vi "Initialize Control.vi"(8 "error in (no error)":errorcluster, 11 "ScrollZoomGraphChart in":refnum<class "ScrollZoomGraphChart.lvclass">=refnum) -> (0 "error out":errorcluster, 3 "ScrollZoomGraphChart out":refnum<class "ScrollZoomGraphChart.lvclass">)   [LabVIEW 2023, in "ScrollZoomGraphChart.lvclass"]
doc: "The <b>Initialize VI</b> is a dynamic dispatch VI that must be overwritten in every QControl Class. It must <b>Call Parent Method</b> so that it recursively calls the initialize routine all of the way up the inheritance hierarchy. \n\nThe top most call is to the <b>Initialize Control VI</b> in Control.lvclass. This is the VI that starts the <b>Event Handler VI</b> if there was one overwritten in the QControl.\n<b> </b> <b> </b>\n©2016 Q Software Innovations, LLC (QSI)\nwritten by Quentin Alldredge\nproduced in LabVIEW 2015\n\nsupport@qsoftwareinnovations.com\nwww.qsoftwareinnovations.com\n\nAll rights reserved.\n\nRedistribution and use in source and binary forms, with or without modification, are permitted provided that the following conditions are met:\n\n * Redistributions of source code must retain the above copyright notice, this list of conditions and the following disclaimer.\n * Redistributions in binary form must reproduce the above copyright notice, this list of conditions and the following disclaimer in the documentation and/or other materials provided with the distribution.\n * Neither the name of Q Software Innovations, LLC. nor the names of its contributors may be used to endorse or promote products derived from this software without specific prior written permission.\n\nTHIS SOFTWARE IS PROVIDED BY THE COPYRIGHT HOLDERS AND CONTRIBUTORS \"AS IS\" AND ANY EXPRESS OR IMPLIED WARRANTIES, INCLUDING, BUT NOT LIMITED TO, THE IMPLIED WARRANTIES OF MERCHANTABILITY AND FITNESS FOR A PARTICULAR PURPOSE ARE DISCLAIMED. IN NO EVENT SHALL THE COPYRIGHT OWNER OR CONTRIBUTORS BE LIABLE FOR ANY DIRECT, INDIRECT, INCIDENTAL, SPECIAL, EXEMPLARY, OR CONSEQUENTIAL DAMAGES (INCLUDING, BUT NOT LIMITED TO, PROCUREMENT OF SUBSTITUTE GOODS OR SERVICES; LOSS OF USE, DATA, OR PROFITS; OR BUSINESS INTERRUPTION) HOWEVER CAUSED AND ON ANY THEORY OF LIABILITY, WHETHER IN CONTRACT, STRICT LIABILITY, OR TORT (INCLUDING NEGLIGENCE OR OTHERWISE) ARISING IN ANY WAY OUT OF THE USE OF THIS SOFTWARE, EVEN IF ADVISED OF THE POSSIBILITY OF SUCH DAMAGE."
uses:
  ScrollZoomGraphChart.lvclass
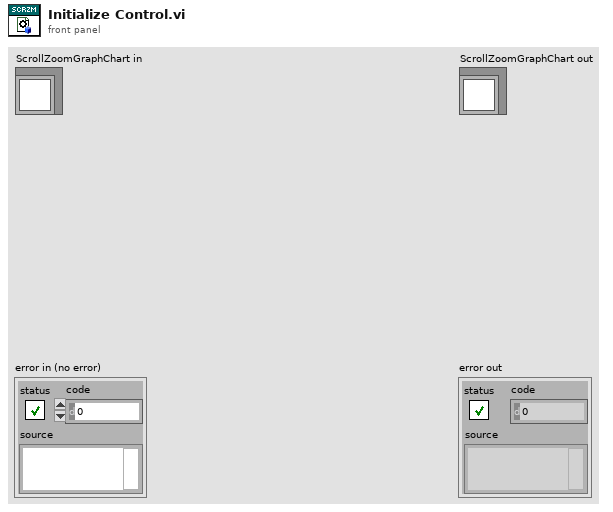
[diagram p1: front panel]
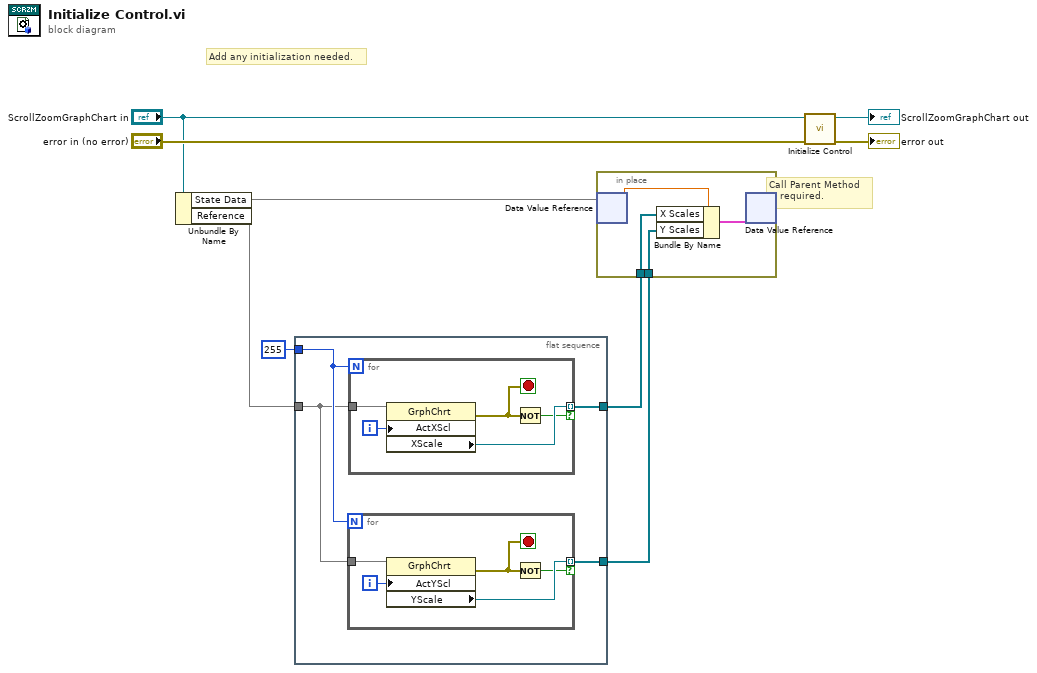
[diagram p0: block diagram]
diagram:
  # "Add any initialization needed."
  # "Call Parent Method\nis required."
  n1 = Unbundle By Name("ScrollZoomGraphChart in") -> ("State Data"=w5, "Reference"=w3)
  n2 = flat-sequence {
    tunnel: [w13] -> w2
    tunnel: [w12] -> w1
    tunnel: 255 -> [w11]
    tunnel: w3 -> [w10]
    frame #0 {
      n3 = for {
        N: w11 -> [_]
        tunnel: w10 -> [w23]
        tunnel: [w21] -> w12 mode=indexing if=w19
        i -> [w22]
        stop <- w20 stop-if-true
        n4 = property class="GrphChrt"(reference=w23, "ActYScl"=w22) -> (error out=w20:errorcluster, "YScale"=w21:refnum<vi>)  [unwired: 1 in, 1 out]
        n5 = Not(x=w20) -> (.not. x?=w19:bool)
      }
      n6 = for {
        N: w11 -> [_]
        tunnel: w10 -> [w18]
        tunnel: [w16] -> w13 mode=indexing if=w14
        i -> [w17]
        stop <- w15 stop-if-true
        n7 = property class="GrphChrt"(reference=w18, "ActXScl"=w17) -> (error out=w15:errorcluster, "XScale"=w16:refnum<vi>)  [unwired: 1 in, 1 out]
        n8 = Not(x=w15) -> (.not. x?=w14:bool)
      }
    }
  }
  n9 = in-place {
    in-place-border: w2 -> [w25]
    in-place-border: w1 -> [w24]
    n10 = in-place-dvr #1(w5) -> (w27:dbl)  [unwired: 1 out]
    n11 = Bundle By Name(cluster=w27, "X Scales"=w25, "Y Scales"=w24) -> (w26:cluster{})
    n12 = in-place-dvr #1(w26) -> ()  [unwired: 2 out]
  }
  n13 = call-parent "Initialize Control.vi"("error in (no error)"="error in (no error)", "Control in"="ScrollZoomGraphChart in") -> ("error out"=→"error out":errorcluster, "Control out"=→"ScrollZoomGraphChart out":refnum<class "ScrollZoomGraphChart.lvclass">)  [unwired: 8 in]
